vi "Open.vi"(0 "SerialPortRef":T2, 5 "UpdateRate (100Hz)":u8=100, 9 "Nav6Mode (YPR)":T3, 11 "error in (no error)":errorcluster) -> (3 "Output Rate (hz)":u32, 4 "Nav6DevRef":T1, 6 "CalibrationState":T4, 8 "Gyroscope Full Scale Range (deg/sec)":u32, 10 "Accelerometer Full Scale Range (g)":u32, 14 "Open Succesfull":bool, 15 "error out":errorcluster)   [LabVIEW 2015, in "Nav6.lvlib"]
doc: "Open a reference to the Nav6 IMU. A reference to a serial port is required to be passed in.\n\nOnly YPR Mode is supported at this time. The Open VI should be placed in Begin in the FRC Framework."
uses:
  Nav6.lvlib
  <vilib>/Rock Robotics/WPI/SerialPort/WPI_SerialPortRef.ctl
  Nav6Mode.ctl
  CalibrationState.ctl
  Nav6DevRef.ctl
  StopGlobal.vi
  <vilib>/Instr/_visa.llb/VISA Configure Serial Port (Instr).vi
panel:
  out "Calibrated Yaw Offset (deg)":dbl
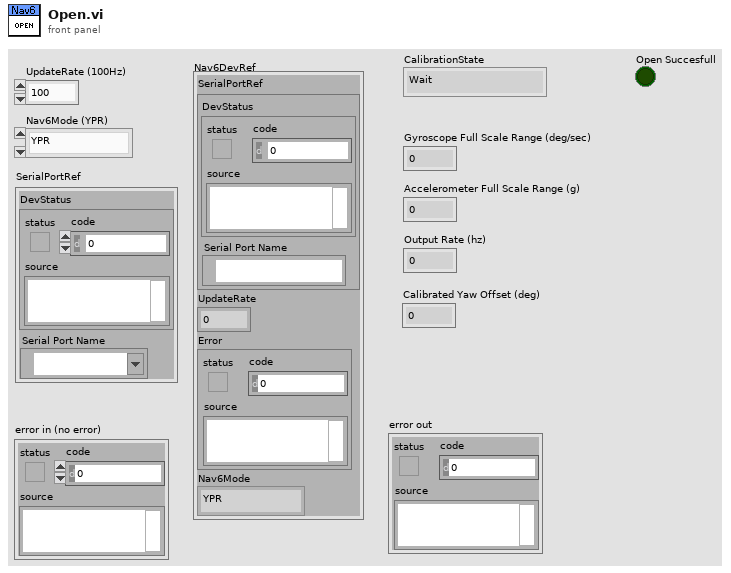
[diagram p1: front panel]
types:
  T1 = typedef "Nav6.lvlib/Nav6DevRef.ctl" = cluster{"SerialPortRef":T2, "UpdateRate":u8, "Error":errorcluster, "Nav6Mode":T3}
  T2 = typedef "WPI_SerialPortRef.ctl" = cluster{"DevStatus":errorcluster, "Serial Port Name":refnum<visa-resource-name>}
  T3 = typedef "Nav6.lvlib/Nav6Mode.ctl" = enum16{"YPR", "Gyro", "Quaternion"}
  T4 = typedef "Nav6.lvlib/CalibrationState.ctl" = enum16{"Wait", "Accumulate", "Complete"}
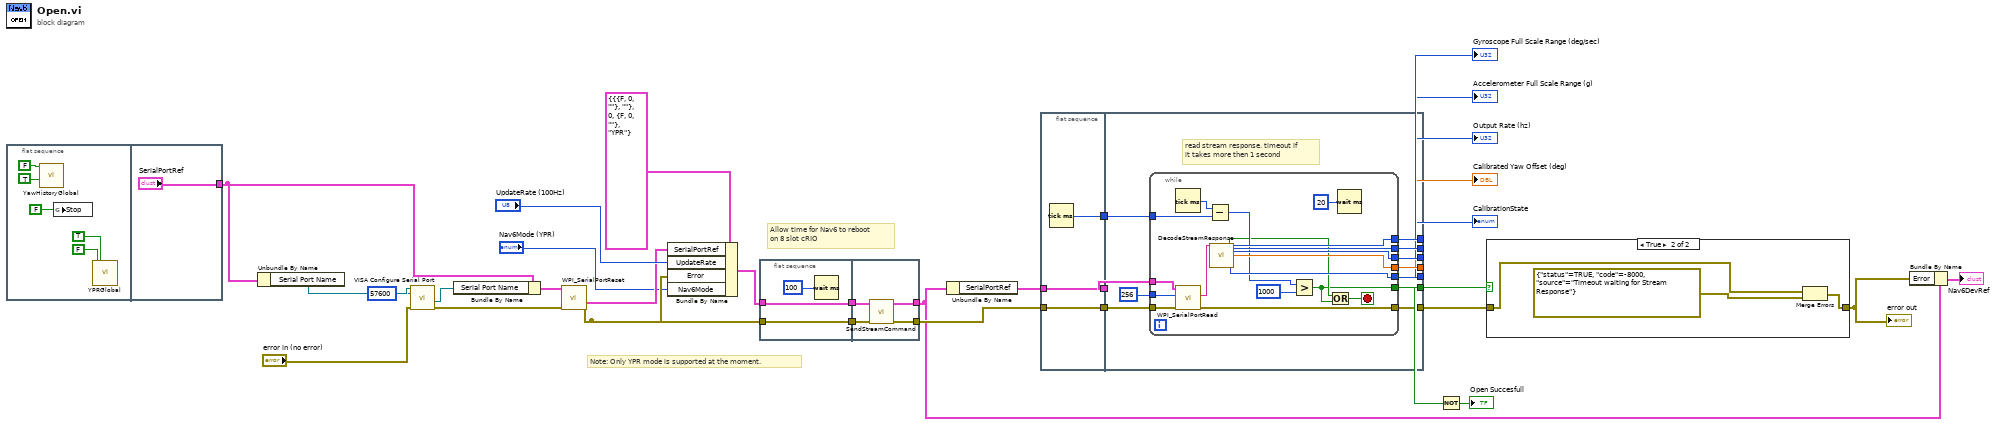
[diagram p0: block diagram]
diagram:
  # "Allow time for Nav6 to reboot\non 8 slot cRIO"
  # "Note: Only YPR mode is supported at the moment."
  n1 = flat-sequence {
    tunnel: ["SerialPortRef"] -> w10
    frame #0 {
      n2 = call "YawHistoryGlobal.vi"("Initialize"=TRUE, "Update"=FALSE) -> ()  [unwired: 9 in, 1 out]
      n3 = global write "StopGlobal.vi" "Stop"(FALSE ("Stop")) -> ()
      n4 = call "YPRGlobal.vi"("Update"=FALSE, "Initialize"=TRUE) -> ()  [unwired: 19 in, 7 out]
    }
    frame #1 {
    }
  }
  n5 = Unbundle By Name(w10) -> ("Serial Port Name"=w26:refnum<visa-resource-name>)
  n6 = call-poly "VISA Configure Serial Port"("VISA resource name"=w26, "baud rate (9600)"=u32 57600, "error in (no error)"="error in (no error)") -> ("VISA resource name out"=w24:refnum<visa-resource-name>, "error out"=w21:errorcluster)  [unwired: 11 in]
  n7 = Bundle By Name(cluster=w10, "Serial Port Name"=w24) -> (w23:T2)
  n8 = call <vilib>:"WPI_SerialPortReset.vi"("error in (no error)"=w21, "SerialPortRef"=w23) -> ("error out"=w28:errorcluster, "SerialPortRef"=w27:T2)  [unwired: 8 in]
  n9 = Bundle By Name(cluster=T1 {"SerialPortRef"={"DevStatus"={"status"=FALSE, "code"=0, "source"=""}, "Serial Port Name"=""}, "UpdateRate"=0, "Error"={"status"=FALSE, "code"=0, "source"=""}, "Nav6Mode"=enum."YPR"} ("Nav6DevRef"), "SerialPortRef"=w27, "UpdateRate"="UpdateRate (100Hz)", "Error"=w28, "Nav6Mode"="Nav6Mode (YPR)") -> (w30:T1)
  n10 = flat-sequence {
    tunnel: w28 -> [w39]
    tunnel: w30 -> [w40]
    tunnel: [w40] -> w2
    tunnel: [w39] -> w1
    tunnel: [w42] -> w14
    tunnel: [w41] -> w7
    tunnel: w2 -> [w44]
    tunnel: w1 -> [w43]
    frame #0 {
      n11 = Wait (ms)(milliseconds to wait=u32 100) -> ()  [unwired: 1 out]
    }
    frame #1 {
      n12 = call "SendStreamCommand.vi"("error in (no error)"=w43, "Nav6DevRef"=w44) -> ("error out"=w42:errorcluster, "Nav6DevRef"=w41:T1)  [unwired: 8 in]
    }
  }
  n13 = Unbundle By Name(w7) -> ("SerialPortRef"=w15:T2)
  n14 = flat-sequence {
    tunnel: w14 -> [w46]
    tunnel: w15 -> [w47]
    tunnel: [w47] -> w6
    tunnel: [w46] -> w5
    tunnel: [w45] -> w4
    tunnel: [w58] -> w20
    tunnel: [w57] -> w19
    tunnel: [w56] -> w18
    tunnel: [w55] -> w17
    tunnel: [w51] -> w13
    tunnel: [w50] -> w12
    tunnel: [w49] -> w11
    tunnel: w6 -> [w54]
    tunnel: w5 -> [w53]
    tunnel: w4 -> [w48]
    frame #0 {
      n15 = Tick Count (ms)() -> (millisecond timer value=w45:u32)
    }
    frame #1 {
      # "read stream response. timeout if\nit takes more then 1 second"
      n16 = while {
        tunnel: [w76] -> w58
        tunnel: [w75] -> w57
        tunnel: [w74] -> w56
        tunnel: [w73] -> w55
        tunnel: [w72] -> w50
        tunnel: w54 -> [w71]
        tunnel: w53 -> [w70]
        tunnel: u32 256 ("Num Bytes to Read") -> [w68]
        tunnel: [w67] -> w51
        tunnel: w48 -> [w61]
        tunnel: [w60] -> w49
        stop <- w63 stop-if-true
        n17 = Tick Count (ms)() -> (millisecond timer value=w62:u32)
        n18 = call <vilib>:"WPI_SerialPortRead.vi"("error in (no error)"=w70, "Num Bytes to Read"=w68, "SerialPortRef"=w71) -> ("error out"=w72:errorcluster, "Buffer"=w69:string)  [unwired: 6 in, 1 out]
        n19 = Subtract(x=w62, y=w61) -> (x-y=w66:u32)
        n20 = call "DecodeStreamResponse.vi"("Buffer"=w69) -> ("ChecksumVerified"=w64:bool, "Flags"=w67:u32, "Gyroscope Full Scale Range"=w76:u32, "Accelerometer Full Scale Range"=w75:u32, "Output Rate"=w74:u32, "Calibrated Yaw Offset"=w73:dbl)  [unwired: 17 in, 4 out]
        n21 = Greater?(x=w66, y=u32 1000) -> (0:w60:bool)
        n22 = Or(x=w64, y=w60) -> (x .or. y?=w63:bool)
        n23 = Wait (ms)(milliseconds to wait=u32 20) -> ()  [unwired: 1 out]
      }
    }
  }
  n24 = Not(x=w11) -> (.not. x?=→"Open Succesfull":bool)
  n25 = case shown="True" w11 {
    tunnel: w12 -> [w77 w80]
    tunnel: [w77 w79] -> w8
    frame False {
    }
    frame True {
      n26 = Merge Errors(w80, errorcluster {"status"=TRUE, "code"=-8000, "source"="Timeout waiting for Stream Response"} ("error in")) -> (w79:errorcluster)
    }
  }
  "error out" <- w8
  n27 = Bundle By Name(cluster=w7, "Error"=w8) -> (→"Nav6DevRef":T1)
  "Calibrated Yaw Offset (deg)" <- w17
  "Output Rate (hz)" <- w18
  "Accelerometer Full Scale Range (g)" <- w19
  "Gyroscope Full Scale Range (deg/sec)" <- w20
  "CalibrationState" <- w13
